vi "Test_Calib.vi"() -> ()   [LabVIEW 2019]
panel:
  out "output array":dbl[](array[numeric])
  in  "array":dbl[](array[numeric])
  in  "Home to top cup locations":dbl[](array[numeric])
  out "Insert name 2":enum16{"Insert #1", "Insert #2", "Calib insert"}(ring)
  out "Lifter locations array_Cal":dbl[](array[numeric])
  out "Lifter locations array_ Calib":dbl[](array[numeric])
  out "Adjusted":dbl[](array[numeric])
  out "adj2":dbl[](array[numeric])
  out "diff 2":dbl
  out "Diff 1":dbl
  in  "Insert name":enum16{"Insert #1", "Insert #2", "Calib insert"}(ring)
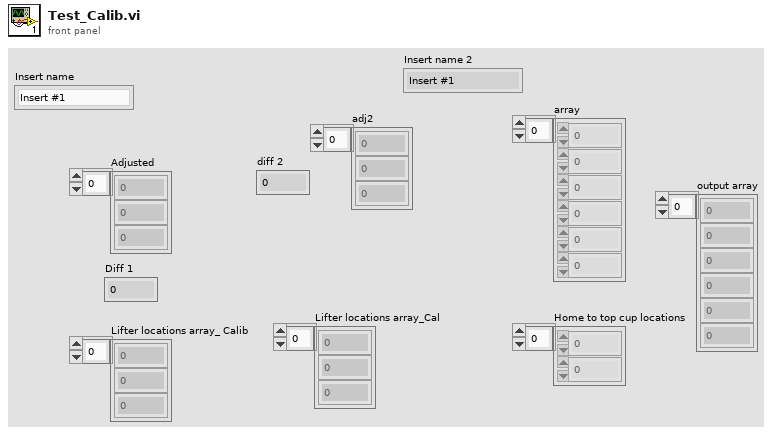
[diagram p1: front panel]
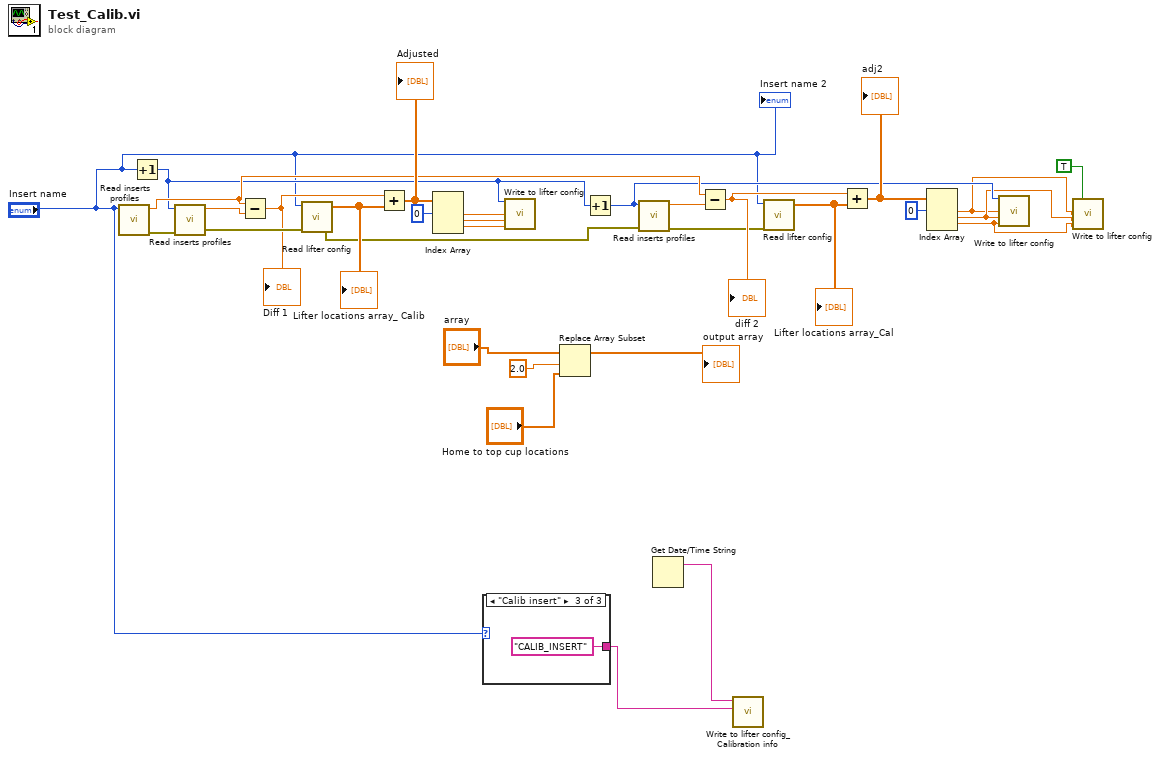
[diagram p0: block diagram]
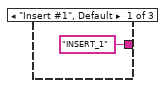
[diagram p2: hidden frame]
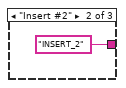
[diagram p3: hidden frame]
diagram:
  n1 = call "Read inserts profiles.vi"("Insert name"="Insert name") -> ("error out"=w31:errorcluster, "top cup length"=w17:dbl)  [unwired: 7 in]
  n2 = Increment(x="Insert name") -> (x+1=w15:enum16{"Insert #1", "Insert #2", "Calib insert"})
  n3 = call "Read inserts profiles.vi"("error in (no error)"=w31, "Insert name"=w15) -> ("error out"=w29:errorcluster, "top cup length"=w30:dbl)  [unwired: 6 in]
  n4 = Subtract(x=w17, y=w30) -> (x-y=w27:dbl)
  "Diff 1" <- w27
  n5 = call "Read lifter config.vi"("Insert name"="Insert name", "error in (no error)"=w29) -> ("Lifter locations array"=w28:dbl[], "error out"=w19:errorcluster)  [unwired: 5 in]
  "Lifter locations array_ Calib" <- w28
  n6 = Add(x=w27, y=w28) -> (x+y=w26:dbl[])
  "Adjusted" <- w26
  n7 = Index Array(array=w26, index #1=0 ("index")) -> (element #1=w25:dbl, element #2=w24:dbl, element #3=w23:dbl)  [unwired: 2 in]
  n8 = case shown="\"Calib insert\"" "Insert name" {
    tunnel: ["INSERT_1" ("section") "INSERT_2" ("section") "CALIB_INSERT" ("section")] -> w2
    frame "Insert #1", Default {
    }
    frame "Insert #2" {
    }
    frame "Calib insert" {
    }
  }
  n9 = call "Write to lifter config.vi"("Insert name"=w15, "Bottom"=w25, "Middle"=w24, "Top"=w23) -> ()  [unwired: 10 in, 2 out]
  n10 = Replace Array Subset(array="array", new element="Home to top cup locations", index=2.0 ("x")) -> (→"output array":dbl[])
  n11 = Increment(x=w15) -> (x+1=w12:enum16{"Insert #1", "Insert #2", "Calib insert"})
  n12 = call "Read inserts profiles.vi"("error in (no error)"=w19, "Insert name"=w12) -> ("error out"=w18:errorcluster, "top cup length"=w22:dbl)  [unwired: 6 in]
  n13 = Get Date/Time String() -> (date string=w3:string)  [unwired: 3 in, 1 out]
  n14 = Subtract(x=w17, y=w22) -> (x-y=w20:dbl)
  "diff 2" <- w20
  n15 = call "Write to lifter config_Calibration info.vi"("Insert"=w2, "Date"=w3) -> ()  [unwired: 7 in, 1 out]
  n16 = call "Read lifter config.vi"("Insert name"="Insert name", "error in (no error)"=w18) -> ("Lifter locations array"=w21:dbl[])  [unwired: 5 in, 1 out]
  "Lifter locations array_Cal" <- w21
  n17 = Add(x=w20, y=w21) -> (x+y=w16:dbl[])
  "adj2" <- w16
  n18 = Index Array(array=w16, index #1=0 ("index")) -> (element #1=w8:dbl, element #2=w9:dbl, element #3=w10:dbl)  [unwired: 2 in]
  n19 = call "Write to lifter config.vi"("Insert name"=w12, "Bottom"=w8, "Middle"=w9, "Top"=w10) -> ()  [unwired: 10 in, 2 out]
  n20 = call "Write to lifter config.vi"("Default"=TRUE, "Bottom"=w8, "Middle"=w9, "Top"=w10) -> ()  [unwired: 10 in, 2 out]
  "Insert name 2" <- "Insert name"
